vi "LEP_RV_BinarySearch.vi"(10 "x":string, 11 "Array":string[](array[string])) -> (3 "Indicate if found x in Array":bool)   [LabVIEW 2011]
panel:
  in  "Start":i32
  in  "End":i32
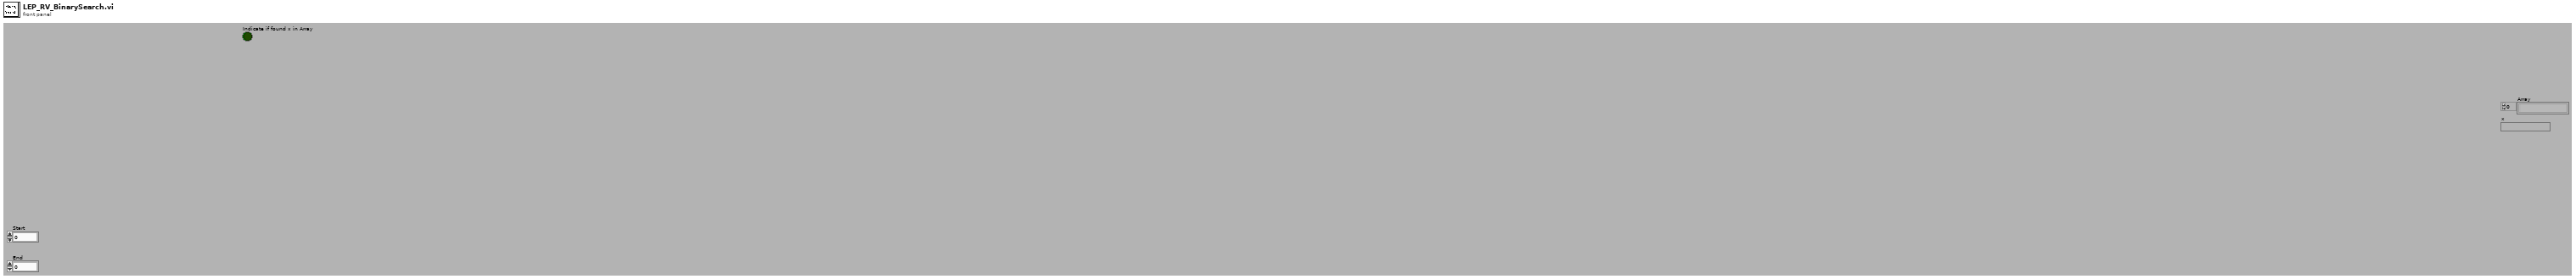
[diagram p1: front panel]
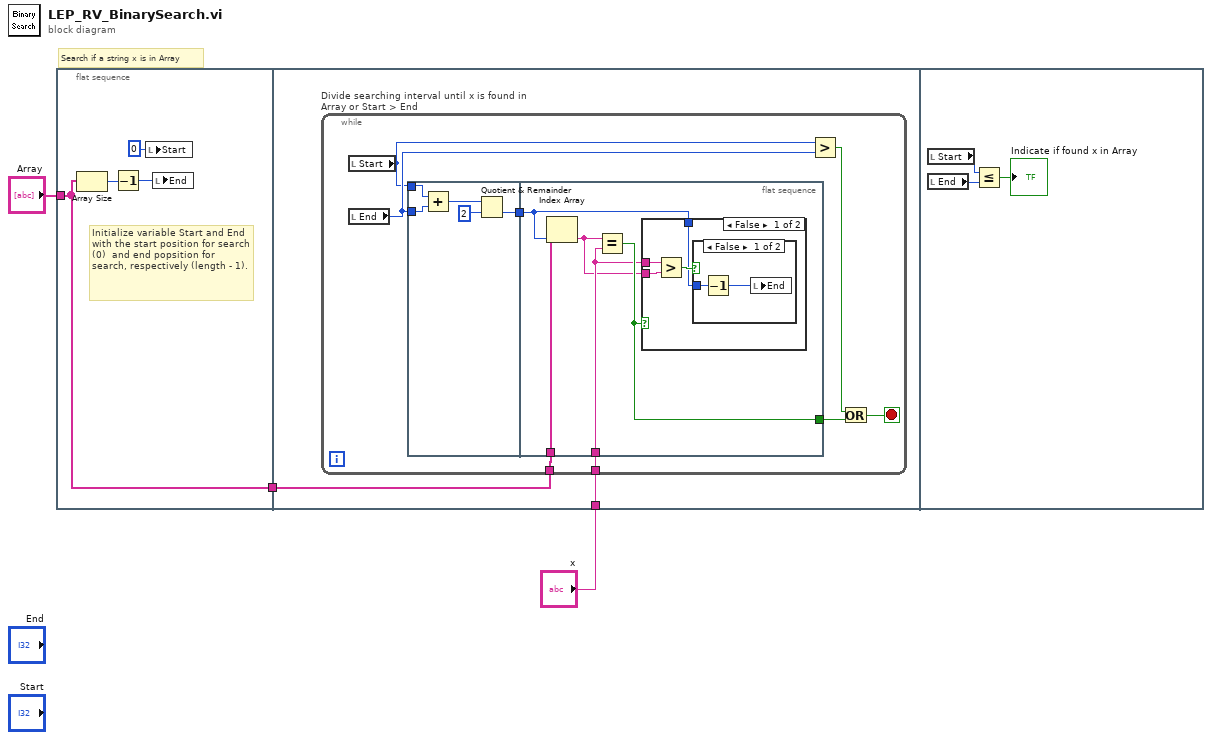
[diagram p0: block diagram]
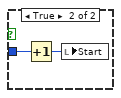
[diagram p2: hidden frame]
diagram:
  # "Search if a string x is in Array"
  n1 = flat-sequence {
    tunnel: "Array" -> [w4]
    tunnel: [w4] -> w3
    tunnel: w3 -> [w8]
    tunnel: "x" -> [w9]
    frame #0 {
      # "Initialize variable Start and End with the start position for search (0)  and end popsition for search, respectively (length - 1)."
      n2 = Array Size(array=w4) -> (size(s)=w6:i32)
      n3 = Decrement(x=w6) -> (x-1=w7:i32)
      n4 = local write "Start"(0 ("Start")) -> ()
      n5 = local write "End"(w7) -> ()
    }
    frame #1 {
      n6 = while "Divide searching interval until x is found in Array or Start > End" {
        tunnel: w9 -> [w11]
        tunnel: w8 -> [w10]
        stop <- w12 stop-if-true
        n7 = local read "Start"() -> (w16:i32)
        n8 = local read "End"() -> (w17:i32)
        n9 = flat-sequence {
          tunnel: w17 -> [w18]
          tunnel: w16 -> [w19]
          tunnel: [w20] -> w15
          tunnel: w15 -> [w25]
          tunnel: [w27] -> w13
          tunnel: w11 -> [w24]
          tunnel: w10 -> [w26]
          frame #0 {
            n10 = Add(x=w19, y=w18) -> (x+y=w22:i32)
            n11 = Quotient & Remainder(x=w22, y=2) -> (floor(x/y)=w20:i32)  [unwired: 1 out]
          }
          frame #1 {
            n12 = Index Array(array=w26, index=w25) -> (element=w23:string)
            n13 = Equal?(x=w23, y=w24) -> (x = y?=w27:bool)
            n14 = case shown="False" w27 {
              tunnel: w25 -> [w30 _]
              tunnel: w24 -> [w29 _]
              tunnel: w23 -> [w28 _]
              frame False {
                n15 = Greater?(x=w29, y=w28) -> (0:w31:bool)
                n16 = case shown="False" w31 {
                  tunnel: w30 -> [w32 w35]
                  frame False {
                    n17 = Decrement(x=w32) -> (x-1=w33:i32)
                    n18 = local write "End"(w33) -> ()
                  }
                  frame True {
                    n19 = Increment(x=w35) -> (x+1=w34:i32)
                    n20 = local write "Start"(w34) -> ()
                  }
                }
              }
              frame True {
              }
            }
          }
        }
        n21 = Greater?(x=w16, y=w17) -> (0:w14:bool)
        n22 = Or(x=w14, y=w13) -> (x .or. y?=w12:bool)
      }
    }
    frame #2 {
      n23 = local read "Start"() -> (w38:i32)
      n24 = local read "End"() -> (w37:i32)
      n25 = Less Or Equal?(x=w38, y=w37) -> (x <= y?=→"Indicate if found x in Array":bool)
    }
  }
